vi "Check If Output Dir Exisits.vi"(0 "directory info in":T1={"target dir"=path "C:/ADIBitbucket/nists19.0_templateproject/Code Modules/Common/Instrument Control/DCPower", "current dir"=path "C:/ADIBitbucket/nists19.0_templateproject/Code Modules/Common/Instrument Control/DCPower", "output dir"={"base dir"=path "../docs", "image dir"=path "../docs", "html dir"=path "../docs", "md dir"=path "../docs"}, "folder names"=[], "filenames"=[]}, 7 "Initial Call":bool, 11 "error in":errorcluster) -> (4 "directory info out":T1={"target dir"=path "C:/ADIBitbucket/nists19.0_templateproject/Code Modules/Common/Instrument Control/DCPower", "current dir"=path "C:/ADIBitbucket/nists19.0_templateproject/Code Modules/Common/Instrument Control/DCPower", "output dir"={"base dir"=path "../docs", "image dir"=path "../docs", "html dir"=path "../docs", "md dir"=path "../docs"}, "folder names"=[], "filenames"=[]}, 15 "error out":errorcluster)   [LabVIEW 2019, in "MD Generator.lvlib"]
uses:
  MD Generator.lvlib
  Report Path Cluster.ctl
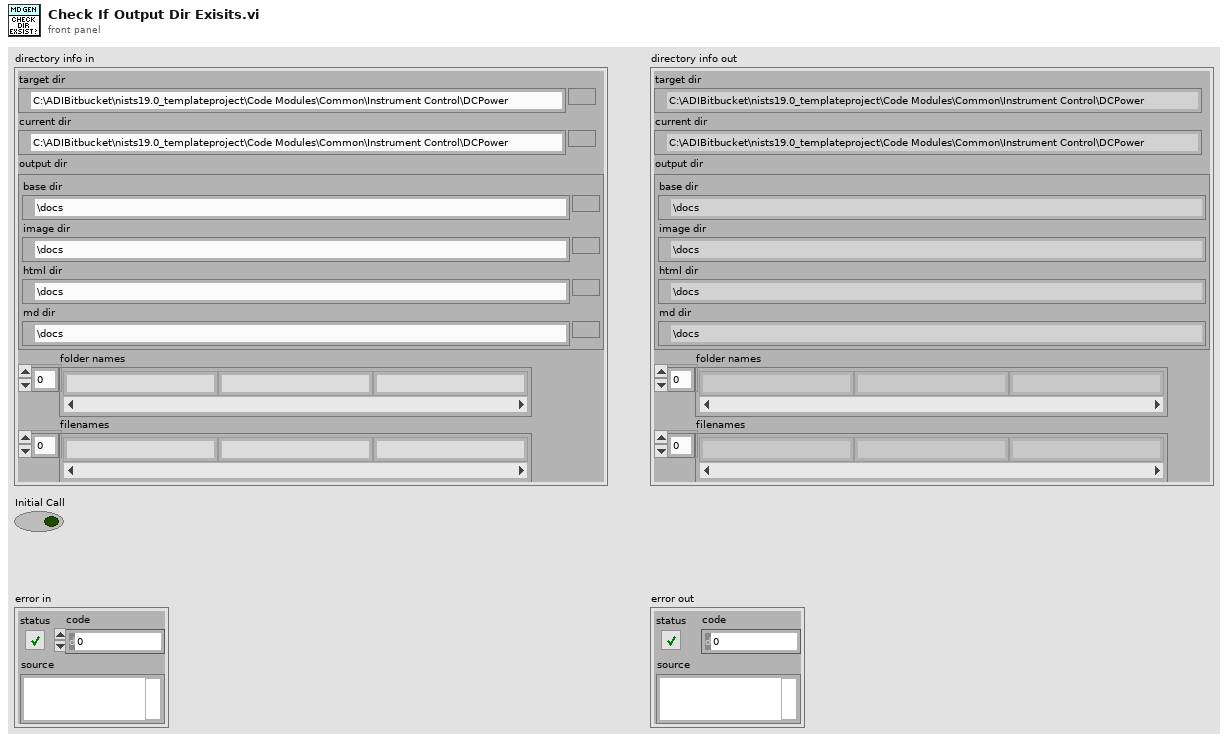
[diagram p1: front panel]
types:
  T1 = typedef "MD Generator.lvlib/Report Path Cluster.ctl" = cluster{"target dir":path, "current dir":path, "output dir":cluster{"base dir":path, "image dir":path, "html dir":path, "md dir":path}, "folder names":string[], "filenames":string[]}
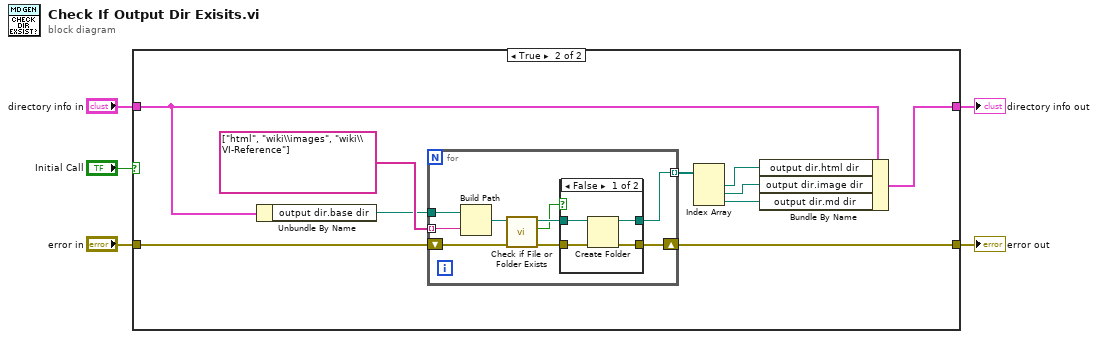
[diagram p0: block diagram]
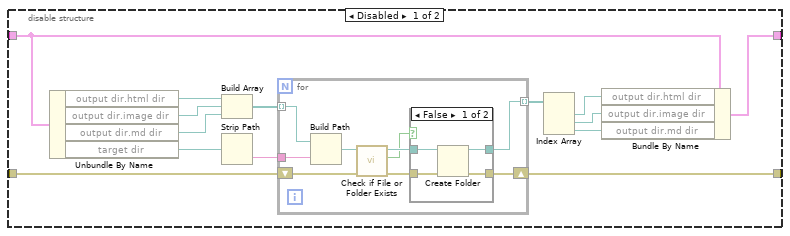
[diagram p3: hidden frame]
diagram:
  n1 = case shown="True" "Initial Call" {
    tunnel: [w7 w50] -> w5
    tunnel: "error in" -> [w6 w48]
    tunnel: "directory info in" -> [w9 w46]
    tunnel: [w8 w45] -> w2
    frame False {
      n2 = disable-structure shown="Enabled" {
        disable-tunnel: w9 -> [w16 w40]
        disable-tunnel: [w15 w40] -> w8
        disable-tunnel: [w14 w39] -> w7
        disable-tunnel: w6 -> [w13 w39]
        frame Disabled {
          n3 = Unbundle By Name(w16) -> ("output dir.html dir"=w23:path, "output dir.image dir"=w22:path, "output dir.md dir"=w21:path, "target dir"=w20:path)
          n4 = Build Array(w23, w22, w21) -> (w11:path[])
          n5 = Strip Path(path=w20) -> (name=w12:string)  [unwired: 1 out]
          n6 = for {
            shift-right: [w30] -> w14
            shift-left: w13 -> [w32]
            tunnel: [w29] -> w19 mode=indexing
            tunnel: w12 -> [w25]
            tunnel: w11 -> [w24] mode=indexing
            n7 = Build Path(base path=w24, name or relative path=w25) -> (appended path=w26:path)
            n8 = call <vilib>:"Check if File or Folder Exists.vi"("error in (no error)"=w32, "path"=w26) -> ("error out"=w31:errorcluster, "file or folder exists?"=w27:bool, "dup path"=w28:path)  [unwired: 7 in]
            n9 = case shown="False" w27 {
              tunnel: w31 -> [w36 w38]
              tunnel: [w35 w38] -> w30
              tunnel: [w34 w37] -> w29
              tunnel: w28 -> [w33 w37]
              frame False {
                n10 = Create Folder(path (use dialog)=w33, error in=w36) -> (created path=w34:path, error out=w35:errorcluster)  [unwired: 1 in, 1 out]
              }
              frame True {
              }
            }
          }
          n11 = Index Array(array=w19) -> (element #1=w10:path, element #2=w18:path, element #3=w17:path)  [unwired: 3 in]
          n12 = Bundle By Name(cluster=w16, "output dir.html dir"=w10, "output dir.image dir"=w18, "output dir.md dir"=w17) -> (w15:T1)
        }
        frame Enabled {
        }
      }
    }
    frame True {
      n13 = Unbundle By Name(w46) -> ("output dir.base dir"=w47:path)
      n14 = for {
        shift-right: [w57] -> w50
        shift-left: w48 -> [w59]
        tunnel: [w56] -> w44 mode=indexing
        tunnel: w47 -> [w52]
        tunnel: string[] ["html", "wiki\\images", "wiki\\VI-Reference"] ("name or relative path") -> [w53] mode=indexing
        n15 = Build Path(base path=w52, name or relative path=w53) -> (appended path=w51:path)
        n16 = call <vilib>:"Check if File or Folder Exists.vi"("error in (no error)"=w59, "path"=w51) -> ("error out"=w58:errorcluster, "file or folder exists?"=w54:bool, "dup path"=w55:path)  [unwired: 7 in]
        n17 = case shown="False" w54 {
          tunnel: w58 -> [w63 w65]
          tunnel: [w62 w65] -> w57
          tunnel: [w61 w64] -> w56
          tunnel: w55 -> [w60 w64]
          frame False {
            n18 = Create Folder(path (use dialog)=w60, error in=w63) -> (created path=w61:path, error out=w62:errorcluster)  [unwired: 1 in, 1 out]
          }
          frame True {
          }
        }
      }
      n19 = Index Array(array=w44) -> (element #1=w43:path, element #2=w42:path, element #3=w41:path)  [unwired: 3 in]
      n20 = Bundle By Name(cluster=w46, "output dir.html dir"=w43, "output dir.image dir"=w42, "output dir.md dir"=w41) -> (w45:T1)
    }
  }
  "error out" <- w5
  "directory info out" <- w2
